vi "Breakpoint - Velocity Equation.vi"() -> ()   [LabVIEW 2020]
uses:
  f1ee70a2-ae65-4fc6-a5ba-ac4ebada8c5b.vi
panel:
  in  "Distance Travelled (s)":dbl
  in  "Constant Acceleration (a)":dbl
  in  "Initial Velocity (u)":dbl
  out "Final Velocity (v)":dbl
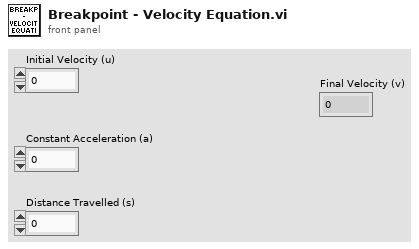
[diagram p1: front panel]
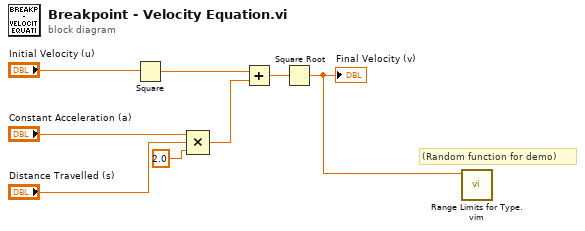
[diagram p0: block diagram]
diagram:
  # "(Random function for demo)"
  n1 = Square(x="Initial Velocity (u)") -> (x^2=w4:dbl)
  n2 = Compound Arithmetic op=MULTIPLY("Constant Acceleration (a)", "Distance Travelled (s)", 2.0 ("value")) -> (w3:dbl)
  n3 = Add(x=w4, y=w3) -> (x+y=w2:dbl)
  n4 = Square Root(x=w2) -> (sqrt(x)=w1:dbl)
  "Final Velocity (v)" <- w1
  n5 = call "Range Limits for Type.vim"("type"=w1) -> ()  [unwired: 9 in, 2 out]
